vi "ADI_IMU_ADIS16448_FGV.vi"(0 "ADI IMU DevRef":T1={"DevStatus"={"status"=FALSE, "code"=0, "source"=""}, "Handle"=0, "SPI Bus"=enum."SPI On-Board, CS0", "Device Found"=FALSE, "Device Ready"=FALSE, "Yaw Axis"=enum."Z", "AHRS Algorithm"=enum."Complementary", "Serial"=0, "Lot ID 2"=0, "Lot ID 1"=0, "Bytes Per Sample"=0, "Calibrate On Open?"=FALSE}, 1 "Operation":enum16{"set", "get", "set reset"}(ring), 2 "Sensor Ready?":bool, 5 "Reset":bool, 7 "IMU Data":T5, 9 "IMU Angles":T3, 11 "IMU AHRS":cluster{"Pitch":dbl, "Roll":dbl, "Yaw":dbl}, 12 "error in":errorcluster) -> (4 "ADI IMU DevRef Out":T1={"DevStatus"={"status"=FALSE, "code"=0, "source"=""}, "Handle"=0, "SPI Bus"=enum."SPI On-Board, CS0", "Device Found"=FALSE, "Device Ready"=FALSE, "Yaw Axis"=enum."Z", "AHRS Algorithm"=enum."Complementary", "Serial"=0, "Lot ID 2"=0, "Lot ID 1"=0, "Bytes Per Sample"=0, "Calibrate On Open?"=FALSE}, 6 "Reset Out":bool, 8 "IMU Data Out":T4, 10 "IMU Angles Out":T3, 13 "Sensor Ready Out":bool, 14 "error out":errorcluster, 15 "IMU AHRS Out":cluster{"Pitch":dbl, "Roll":dbl, "Yaw":dbl})   [LabVIEW 2019, in "ADIS16448_IMU.lvlib"]
uses:
  ADIS16448_IMU.lvlib
  ADI_IMU_ADIS16448_IMUDevRef.ctl
  <vilib>/Rock Robotics/SystemInterfaces/spilib/spi_bus.ctl
panel:
  in  "Offset Compensated Data":dbl[](array[numeric])
  out "Offset Compensated Data Out":dbl[](array[numeric])
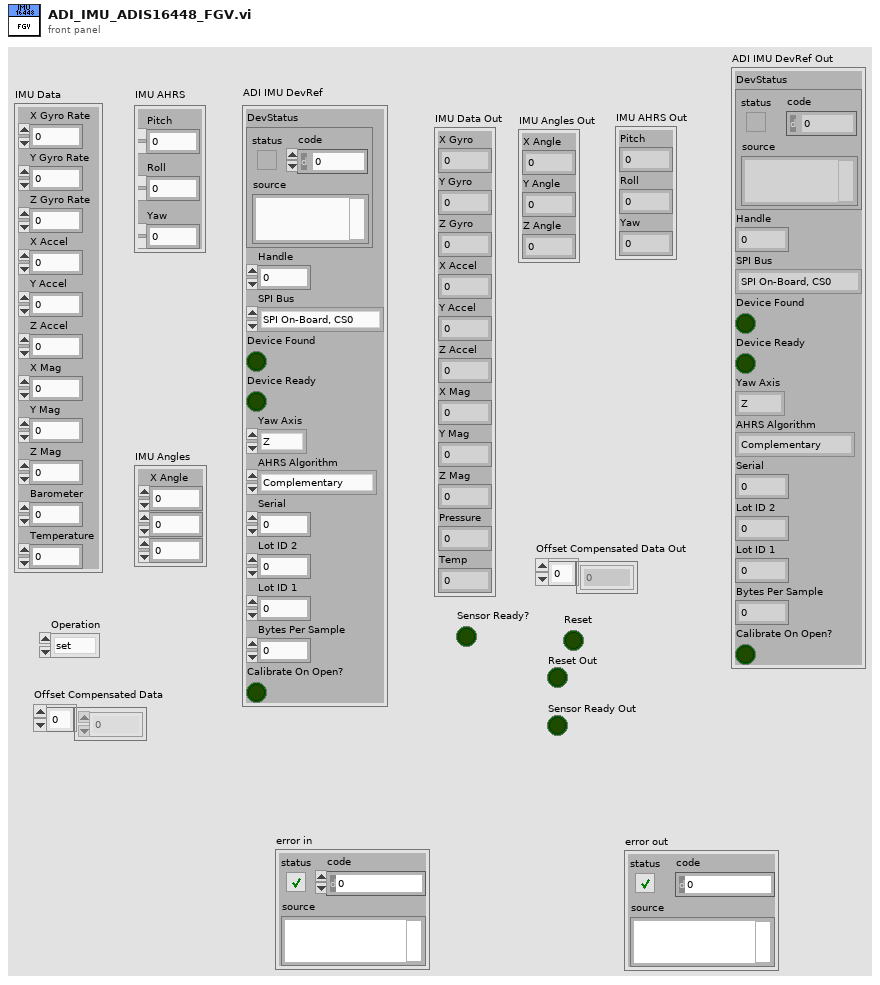
[diagram p1: front panel]
types:
  T1 = typedef "ADIS16448_IMU.lvlib/ADI_IMU_ADIS16448_IMUDevRef.ctl" = cluster{"DevStatus":errorcluster, "Handle":i32, "SPI Bus":T2, "Device Found":bool, "Device Ready":bool, "Yaw Axis":enum16{"X", "Y", "Z"}, "AHRS Algorithm":enum16{"Complementary", "Madgwick"}, "Serial":u16, "Lot ID 2":u16, "Lot ID 1":u16, "Bytes Per Sample":u16, "Calibrate On Open?":bool}
  T2 = typedef "spi_bus.ctl" = enum16{"SPI On-Board, CS0", "SPI On-Board, CS1", "SPI On-Board, CS2", "SPI On-Board, CS3", "SPI MXP", "Invalid"}
  T3 = cluster{"X Angle":dbl, "Y Angle":dbl, "Z Angle":dbl}
  T4 = cluster{"X Gyro":dbl, "Y Gyro":dbl, "Z Gyro":dbl, "X Accel":dbl, "Y Accel":dbl, "Z Accel":dbl, "X Mag":dbl, "Y Mag":dbl, "Z Mag":dbl, "Pressure":dbl, "Temp":dbl}
  T5 = cluster{"X Gyro Rate":dbl, "Y Gyro Rate":dbl, "Z Gyro Rate":dbl, "X Accel":dbl, "Y Accel":dbl, "Z Accel":dbl, "X Mag":dbl, "Y Mag":dbl, "Z Mag":dbl, "Barometer":dbl, "Temperature":dbl}
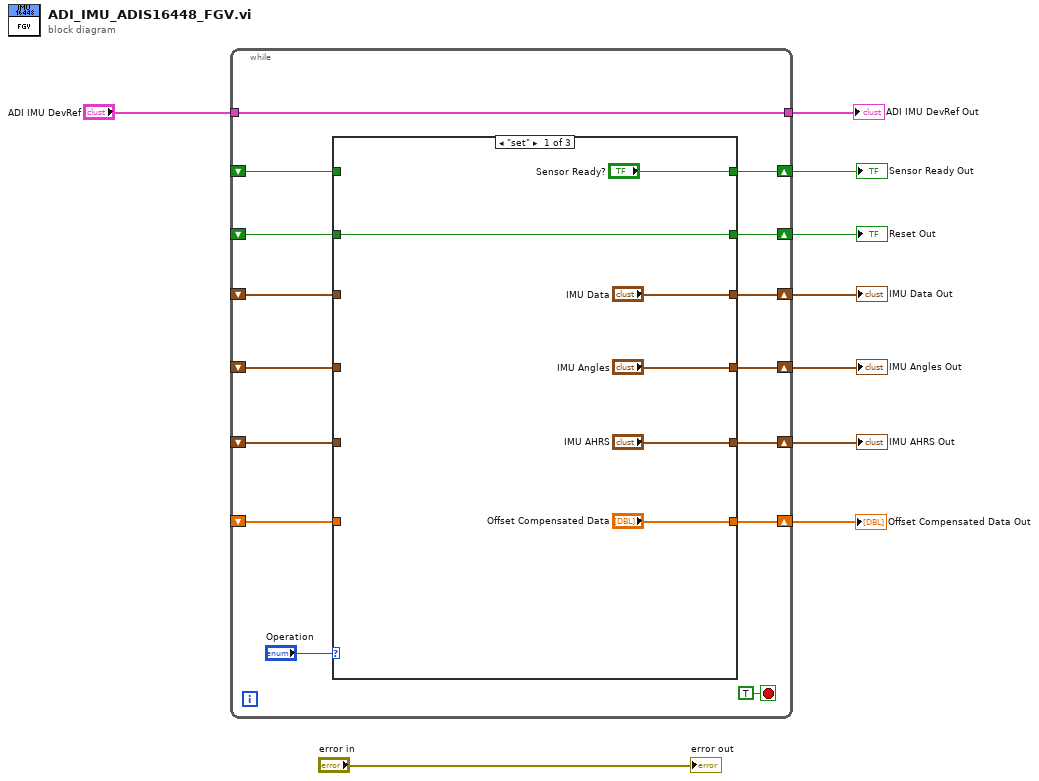
[diagram p0: block diagram]
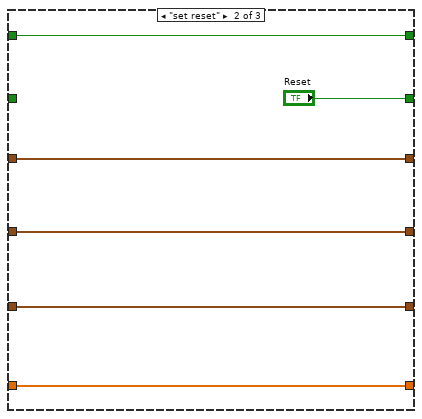
[diagram p2: hidden frame]
diagram:
  n1 = while {
    shift-right: [w22] -> w9
    shift-left: _ -> [w16]
    shift-right: [w21] -> w6
    shift-left: _ -> [w17]
    tunnel: "ADI IMU DevRef" -> [w20]
    tunnel: [w20] -> w7
    shift-right: [w19] -> w5
    shift-left: _ -> [w18]
    shift-right: [w15] -> w4
    shift-left: _ -> [w14]
    shift-right: [w13] -> w2
    shift-left: _ -> [w12]
    shift-right: [w10] -> w8
    shift-left: _ -> [w11]
    stop <- TRUE stop-if-true
    n2 = case shown="\"set\"" "Operation" {
      tunnel: [w26 "Reset" w40] -> w22
      tunnel: ["IMU Data" w32 w41] -> w21
      tunnel: ["IMU Angles" w33 w42] -> w19
      tunnel: w18 -> [_ w33 w42]
      tunnel: w17 -> [_ w32 w41]
      tunnel: w16 -> [w26 _ w40]
      tunnel: ["IMU AHRS" w34 w39] -> w15
      tunnel: w14 -> [_ w34 w39]
      tunnel: ["Offset Compensated Data" w35 w38] -> w13
      tunnel: w12 -> [_ w35 w38]
      tunnel: ["Sensor Ready?" w31 w37] -> w10
      tunnel: w11 -> [_ w31 w37]
      frame "set" {
      }
      frame "set reset" {
      }
      frame "get", Default {
      }
    }
  }
  "Reset Out" <- w9
  "Sensor Ready Out" <- w8
  "IMU Data Out" <- w6
  "IMU Angles Out" <- w5
  "IMU AHRS Out" <- w4
  "ADI IMU DevRef Out" <- w7
  "Offset Compensated Data Out" <- w2
  "error out" <- "error in"
